vi "Get_Rel_Path.vi"(7 "Parrent Folder":path, 8 "error in (no error)":errorcluster, 11 "Source File":path=path "D:/DNN/_from_Customer/2025/2025_05_21_Medtronic_Ireland/1_Dataset/00_Orig") -> (0 "error out":errorcluster, 1 "Rel Path without extension":path, 2 "Rel Path":path, 3 "FIle Dup":path=path "D:/DNN/_from_Customer/2025/2025_05_21_Medtronic_Ireland/1_Dataset/00_Orig")   [LabVIEW 2020]
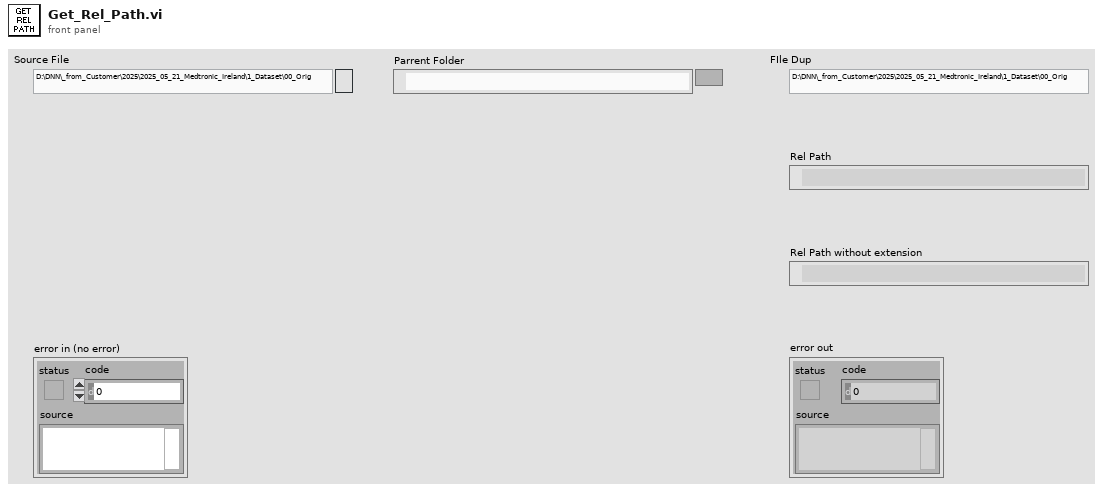
[diagram p1: front panel]
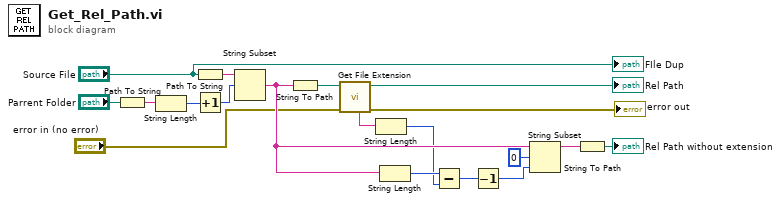
[diagram p0: block diagram]
diagram:
  n1 = Path To String(path="Parrent Folder") -> (string=w19:string)
  n2 = String Length(string=w19) -> (length=w18:i32)
  n3 = Path To String(path="Source File") -> (string=w16:string)
  n4 = Increment(x=w18) -> (x+1=w17:i32)
  n5 = String Subset(string=w16, offset (0)=w17) -> (substring=w8:string)  [unwired: 1 in]
  n6 = String To Path(string=w8) -> (path=w13:path)
  n7 = call <vilib>:"Get File Extension.vi"("error in (no error)"="error in (no error)", "file"=w13) -> ("error out"=→"error out":errorcluster, "dup file"=→"Rel Path":path, "unmodified file extension"=w9:string)  [unwired: 5 in, 2 out]
  n8 = String Length(string=w9) -> (length=w6:i32)
  n9 = String Length(string=w8) -> (length=w7:i32)
  n10 = Subtract(x=w7, y=w6) -> (x-y=w5:i32)
  n11 = Decrement(x=w5) -> (x-1=w3:i32)
  n12 = String Subset(string=w8, offset (0)=0, length (rest)=w3) -> (substring=w10:string)
  n13 = String To Path(string=w10) -> (path=→"Rel Path without extension":path)
  "FIle Dup" <- "Source File"
